vi "Ctor.vi"(8 "error in (no error)":errorcluster, 11 "BP Summary in":refnum<class "BP Summary.lvclass">) -> (0 "error out":errorcluster, 3 "BP Summary out":refnum<class "BP Summary.lvclass">)   [LabVIEW 2020, in "BP Summary.lvclass"]
uses:
  BP Summary.lvclass
  Ref Data.ctl
  BP Summary.lvclass/BP Summary.ctl
  lv-oopanel/OOPanel/ArrayPanel/ArrayPanel.lvclass
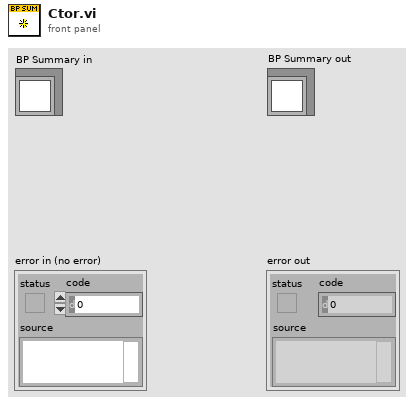
[diagram p1: front panel]
types:
  T1 = typedef "BP Summary.lvclass/Ref Data.ctl" = cluster{"Show Components":bool}
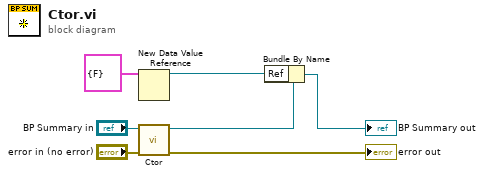
[diagram p0: block diagram]
diagram:
  n1 = New Data Value Reference(data value=T1 {"Show Components"=FALSE} ("Ref Data")) -> (data value reference=w1:refnum<data-value>)  [unwired: 1 in, 1 out]
  n2 = call-parent "Ctor.vi"("error in (no error)"="error in (no error)", "ArrayPanel in"="BP Summary in") -> ("error out"=→"error out":errorcluster, "ArrayPanel out"=w5:refnum<class "BP Summary.lvclass">)  [unwired: 8 in]
  n3 = Bundle By Name(cluster=w5, "Ref"=w1) -> (→"BP Summary out":refnum<class "BP Summary.lvclass">)
